vi "Main On Load Action VI.vi"(8 "error in (no error)":errorcluster, 11 "Device Item Ref in":T1 format="%.0x") -> (0 "error out":errorcluster, 3 "Device Item Ref out":T1 format="%.0x")   [LabVIEW 2020, in "Ballard 1553 System Explorer.lvlib"]
uses:
  Ballard 1553 System Explorer.lvlib
  <vilib>/NI VeriStand/Custom Device API/Custom Device Item Ref.ctl
  <vilib>/NI VeriStand/Custom Device API/Custom Device API.lvlib
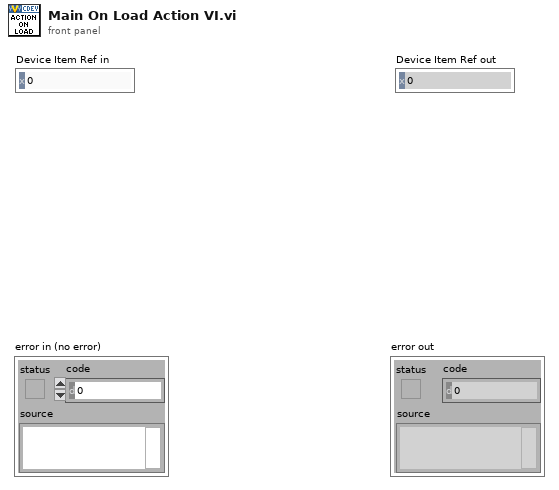
[diagram p1: front panel]
types:
  T1 = typedef "Custom Device API.lvlib/Custom Device Item Ref.ctl" = u64
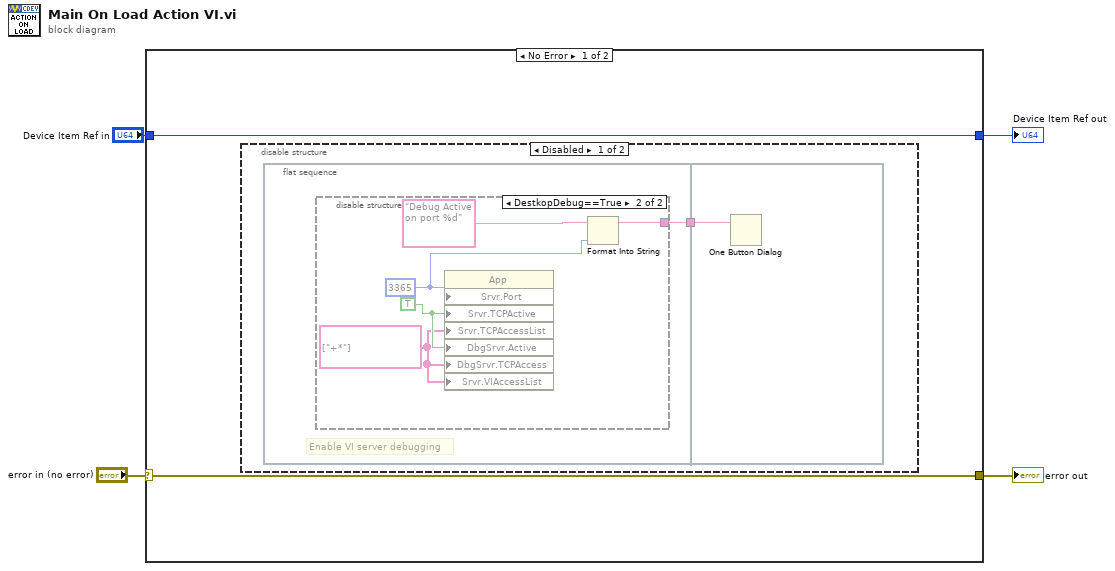
[diagram p0: block diagram]
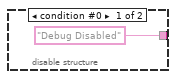
[diagram p2: hidden frame]
diagram:
  n1 = case shown="No Error" "error in (no error)" {
    selector: "error in (no error)" -> [w6 w17]
    tunnel: [w6 w17] -> w3
    tunnel: "Device Item Ref in" -> [w5 w16]
    tunnel: [w5 w16] -> w1
    frame No Error {
      n2 = disable-structure shown="Disabled" {
        frame Disabled {
          n3 = flat-sequence {
            tunnel: [w8] -> w7
            tunnel: w7 -> [w15]
            frame #0 {
              # "Enable VI server debugging"
              n4 = disable-structure shown="DestkopDebug==True" {
                disable-tunnel: ["Debug Disabled" w11] -> w8
                frame condition #0 {
                }
                frame condition #1 (active) {
                  w10 = string[] ["+*"] ("Server:TCP/IP Access List")
                  w14 = TRUE ("Server:TCP Listener Active")
                  w12 = u32 3365 ("Server:Port")
                  n5 = property class="App"("Srvr.Port"=w12, "Srvr.TCPActive"=w14, "Srvr.TCPAccessList"=w10, "DbgSrvr.Active"=w14, "DbgSrvr.TCPAccess"=w10, "Srvr.VIAccessList"=w10) -> ()  [unwired: 2 in, 2 out]
                  n6 = Format Into String(format string="Debug Active on port %d" ("message"), w12) -> (resulting string=w11:string)  [unwired: 2 in, 1 out]
                }
              }
            }
            frame #1 {
              n7 = One Button Dialog(message=w15) -> ()  [unwired: 1 in, 1 out]
            }
          }
        }
        frame Enabled {
        }
      }
    }
    frame Error {
    }
  }
  "error out" <- w3
  "Device Item Ref out" <- w1
